vi "chem dose pump (mLpers).vi"(4 "State":i16, 5 "Time":dbl format="%.2f", 6 "Sensor Values":dbl[](array[numeric]), 7 "Set Points":dbl[](array[numeric])) -> (0 "required data":T2={"Set Point names"=["plant flow (mL/s)", " stock concentration (mg/L)", "desired dose (mg/L)", "tubing size (13, 14, 16, 25, 17, 18)"], "required number of setpoints"=4, "required number of sensors"=0, "Sensor names"=[]}, 3 "output value":dbl)   [LabVIEW 2019]
panel:
  in  "tubing size":enum16{"13", "14", "16", "25", "17", "18"}(ring)
  in  "Pump":T1 {"flow rate" format="%.4f"}
  # "rpm/100"
  # "Enter the correct information for this control code in the required data structure below. Then make the current value default by right clicking on the border of the data structure. Select \"data operations\" and then select \"make current value default\". These values will be displayed by process controller."
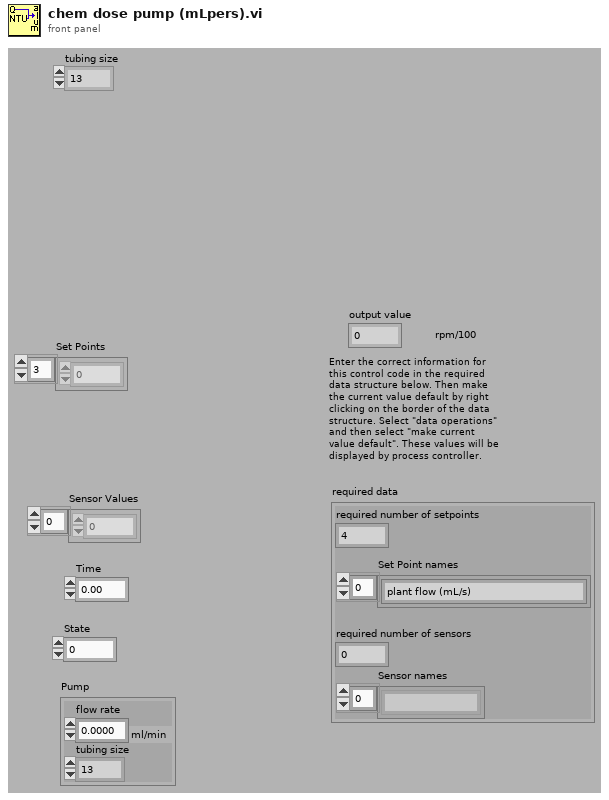
[diagram p1: front panel]
types:
  T1 = cluster{"tubing size":enum16{"13", "14", "16", "25", "17", "18"}, "flow rate":dbl[unit]}
  T2 = cluster{"Set Point names":string[], "required number of setpoints":u8, "required number of sensors":u8, "Sensor names":string[]}
  T3 = cluster{"Set Points[0]":dbl, "Set Points[1]":dbl, "Set Points[2]":dbl, "Set Points[3]":dbl}
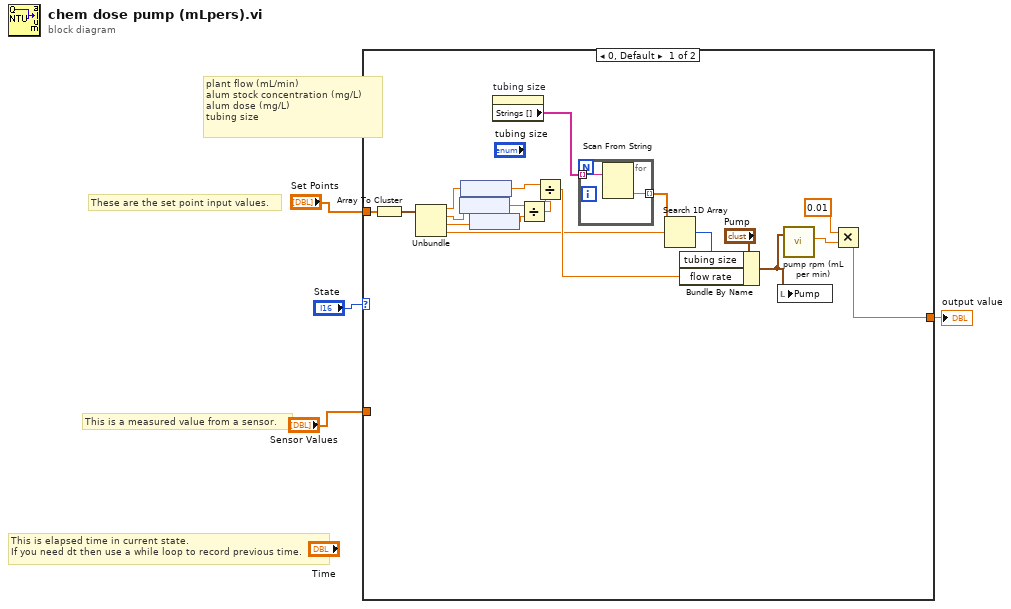
[diagram p0: block diagram]
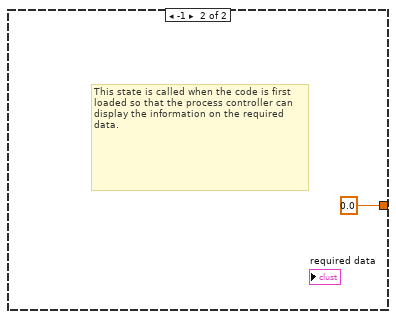
[diagram p2: hidden frame]
diagram:
  # "plant flow (mL/min)\nalum stock concentration (mg/L)\nalum dose (mg/L)\ntubing size"
  # "These are the set point input values."
  # "This is a measured value from a sensor."
  # "This is elapsed time in current state.\nIf you need dt then use a while loop to record previous time."
  n1 = case shown="0, Default" "State" {
    tunnel: [w7 0.0 ("fraction on")] -> w3
    tunnel: "Set Points" -> [w8 _]
    tunnel: "Sensor Values" -> [_ _]
    frame 0, Default {
      n2 = Array To Cluster(array=w8) -> (cluster=w23:T3)
      n3 = Unbundle(w23) -> ("Set Points[0]"=w12:dbl, "Set Points[1]"=w11:dbl, "Set Points[2]"=w10:dbl, "Set Points[3]"=w9:dbl)
      n4 = node(w11) -> (w16:dbl[unit])
      n5 = node(w12) -> (w15:dbl[unit])
      n6 = node(w10) -> (w17:dbl[unit])
      n7 = property on="tubing size" class="Enum (strict)"() -> ("Strings []"=w6:string[])  [unwired: 2 in, 2 out]
      n8 = Divide(x=w16, y=w17) -> (x/y=w14:dbl)
      n9 = Divide(x=w15, y=w14) -> (x/y=w13:dbl[unit])
      n10 = for {
        tunnel: w6 -> [w25] mode=indexing
        tunnel: [w24] -> w22 mode=indexing
        n11 = Scan From String(input string=w25) -> (output 1=w24:dbl)  [unwired: 4 in, 3 out]
      }
      n12 = Search 1D Array(1D array=w22, element=w9) -> (index of element=w20:i32)  [unwired: 1 in]
      n13 = Bundle By Name(cluster="Pump", "tubing size"=w20, "flow rate"=w13) -> (w5:T1)
      n14 = local write "Pump"(w5) -> ()
      n15 = call "pump rpm (mL per min).vi"("Pump"=w5) -> ("pump speed (rpm)"=w19:dbl)  [unwired: 1 in, 3 out]
      n16 = Multiply(x=0.01, y=w19) -> (x*y=w7:dbl)
    }
    frame -1 {
      # "This state is called when the code is first loaded so that the process controller can display the information on the required data."
    }
  }
  "output value" <- w3
